vi "Test HTTP Header Read Timeout.vi"(8 "error in (no error)":errorcluster, 11 "TestCase in":refnum<class "Test WebSockets Core.lvclass">) -> (0 "error out":errorcluster, 3 "TestCase out":refnum<class "Test WebSockets Core.lvclass">)   [LabVIEW 2013, in "Test WebSockets Core.lvclass"]
uses:
  Test WebSockets Core.lvclass
  <vilib>/addons/_JKI Toolkits/VI Tester/TestCase.llb/TestCase.lvclass
  WebSockets/WebSocket/WebSocket.lvclass
  WebSockets/WebSockets.lvlib
panel:
  out "Read time":u32
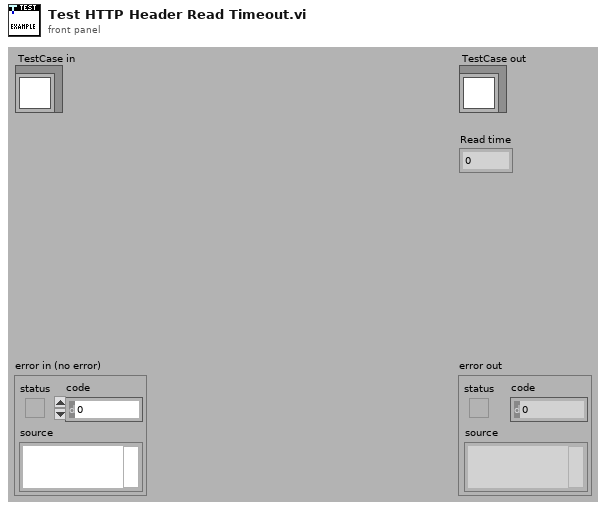
[diagram p1: front panel]
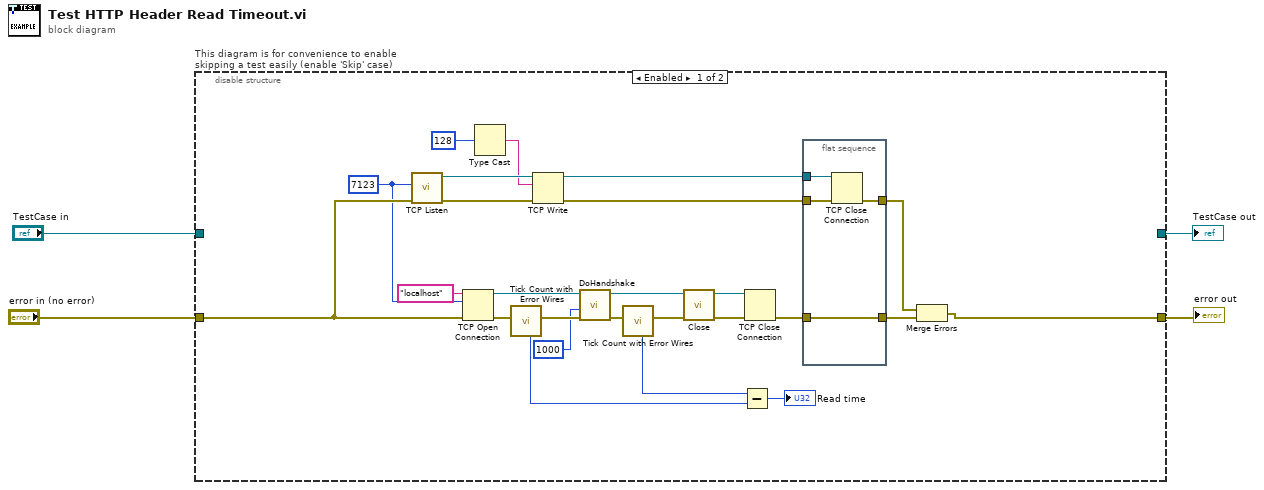
[diagram p0: block diagram]
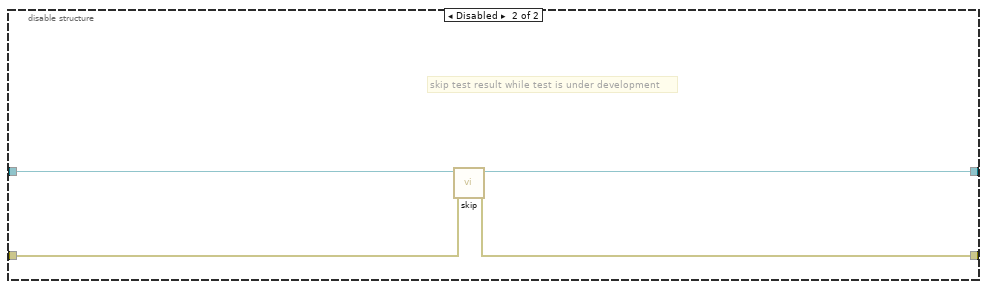
[diagram p2: hidden frame]
diagram:
  n1 = disable-structure "This diagram is for convenience to enable skipping a test easily (enable 'Skip' case)" shown="Enabled" {
    disable-tunnel: "TestCase in" -> [_ w37]
    disable-tunnel: [_ w35] -> w1
    disable-tunnel: [w26 w36] -> w3
    disable-tunnel: "error in (no error)" -> [w29 w34]
    frame Enabled {
      w28 = u16 7123 ("port")
      n2 = call <vilib>:"TCP Listen.vi"("error in (no error)"=w29, "port"=w28) -> ("error out"=w25:errorcluster, "connection ID"=w24:refnum<k5>)  [unwired: 5 in, 3 out]
      n3 = TCP Open Connection(address="localhost", remote port or service name=w28, error in (no error)=w29) -> (connection ID=w10:refnum<k5>, error out=w15:errorcluster)  [unwired: 2 in]
      n4 = Type Cast(x=u8 128) -> (*(type *) &x=w22:string)  [unwired: 1 in]
      n5 = call "Tick Count with Error Wires.vi"("error in (no error)"=w15) -> ("error out"=w11:errorcluster, "millisecond timer value"=w13:u32)  [unwired: 9 in]
      n6 = TCP Write(connection ID=w24, data in=w22, error in (no error)=w25) -> (connection ID out=w17:refnum<k5>, error out=w18:errorcluster)  [unwired: 1 in, 1 out]
      n7 = call "DoHandshake.vi"("error in (no error)"=w11, "timeout ms (5000)"=1000, "TCP Connection in"=w10) -> ("error out"=w9:errorcluster, "WebSocket Server out"=w6:refnum<class "WebSocket Server.lvclass">)  [unwired: 5 in, 2 out]
      n8 = call "Tick Count with Error Wires.vi"("error in (no error)"=w9) -> ("error out"=w16:errorcluster, "millisecond timer value"=w14:u32)  [unwired: 9 in]
      n9 = call "Close.vi"("error in (no error)"=w16, "WebSocket in"=w6) -> ("error out"=w7:errorcluster, "TCP Connection out"=w5:refnum<k5>)  [unwired: 8 in]
      n10 = Subtract(x=w14, y=w13) -> (x-y=→"Read time":u32)
      n11 = TCP Close Connection(connection ID=w5, error in (no error)=w7) -> (error out=w21:errorcluster)  [unwired: 1 in, 1 out]
      n12 = flat-sequence {
        tunnel: w21 -> [w33]
        tunnel: [w33] -> w20
        tunnel: [w32] -> w19
        tunnel: w18 -> [w31]
        tunnel: w17 -> [w30]
        frame #0 {
          n13 = TCP Close Connection(connection ID=w30, error in (no error)=w31) -> (error out=w32:errorcluster)  [unwired: 1 in, 1 out]
        }
      }
      n14 = Merge Errors(w19, w20) -> (w26:errorcluster)
    }
    frame Disabled {
      # "skip test result while test is under development"
      n15 = call <vilib>:"skip.vi"("error in (no error)"=w34, "TestCase in"=w37) -> ("error out"=w36:errorcluster, "TestCase out"=w35:refnum<class "Test WebSockets Core.lvclass">)  [unwired: 8 in]
    }
  }
  "error out" <- w3
  "TestCase out" <- w1
